vi "Sensor de Flujo.vi"() -> ()   [LabVIEW 2015]
uses:
  <vilib>/LabVIEW Interface for Arduino/Type Defs/Connection Type.ctl
  <vilib>/LabVIEW Interface for Arduino/Type Defs/Board Type.ctl
  <vilib>/LabVIEW Interface for Arduino/Type Defs/Pin Mode.ctl
  <vilib>/LabVIEW Interface for Arduino/LabVIEW Interface for Arduino.lvlib
  <vilib>/ptbypt/NI_PtbyPt.lvlib
panel:
  in  "Digital I/O Pin (0)":u8
  in  "VISA resource":refnum<visa-resource-name>
  out "LITROS POR MINUTO":dbl(graph)
  out "Horizontal Graduated Bar":dbl(slide) scale=0.0..100.0
  out "LITROS POR MINUTO 2":dbl(knob) scale=0.0..100.0
  out "Numeric":i32
  out "PULSOS POR SEGUNDO":i32
  out "CONTRO TIEMPO":dbl
  out "CONTEO":i32
  out "?":bool
  out "LITROS POR MINUTO":dbl
  out "?":string
  out "?":bool
  in  "?":bool
  # "MEDICIÓN DE FLUJO ATRAVEZ DEL SENSOR YF-S201"
  # "Militros/min"
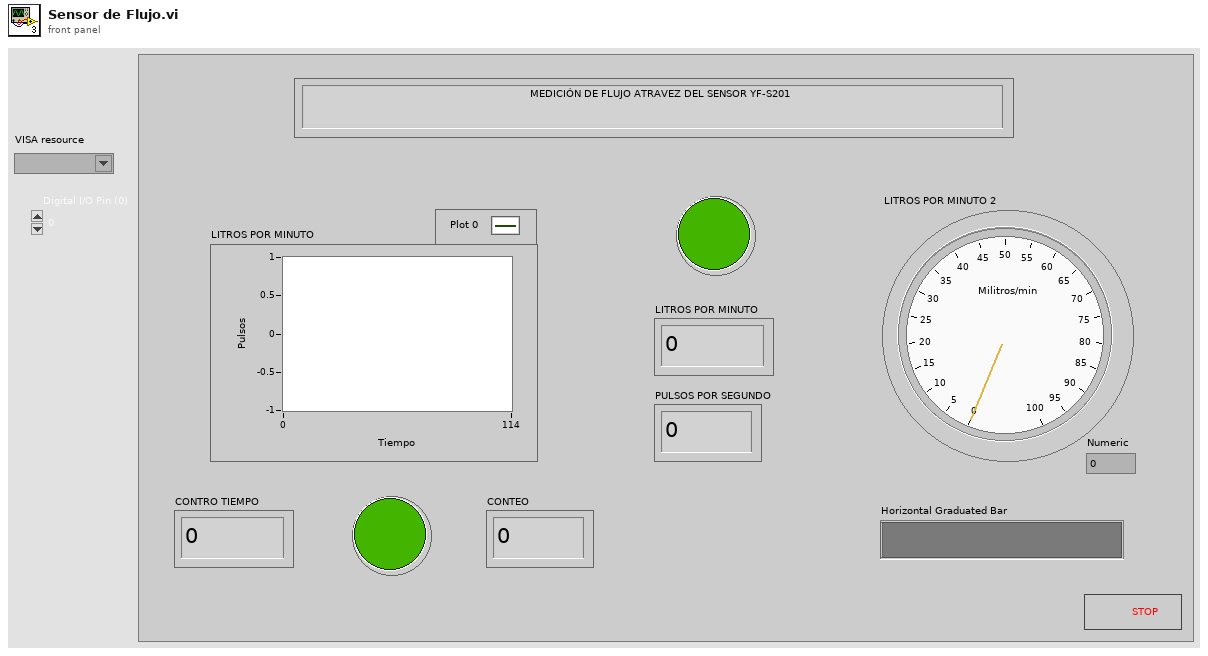
[diagram p1: front panel]
types:
  T1 = typedef "LabVIEW Interface for Arduino.lvlib/Board Type.ctl" = enum16{"Uno", "Dimuelanove w/Atmega 328", "Mega 2560"}
  T2 = typedef "LabVIEW Interface for Arduino.lvlib/Connection Type.ctl" = enum8{"USB / Serial", "XBEE", "BlueSmirf (Bluetooth)"}
  T3 = typedef "LabVIEW Interface for Arduino.lvlib/Arduino Resource.ctl" = cluster{"VISA resource":refnum<visa-resource-name>, "Board Type":T1, "Connection Type":enum8{"USB / Serial"}, "Bytes Per Packet (15)":u8}
  T4 = typedef "LabVIEW Interface for Arduino.lvlib/Pin Mode.ctl" = enum8{"Input", "Output"}
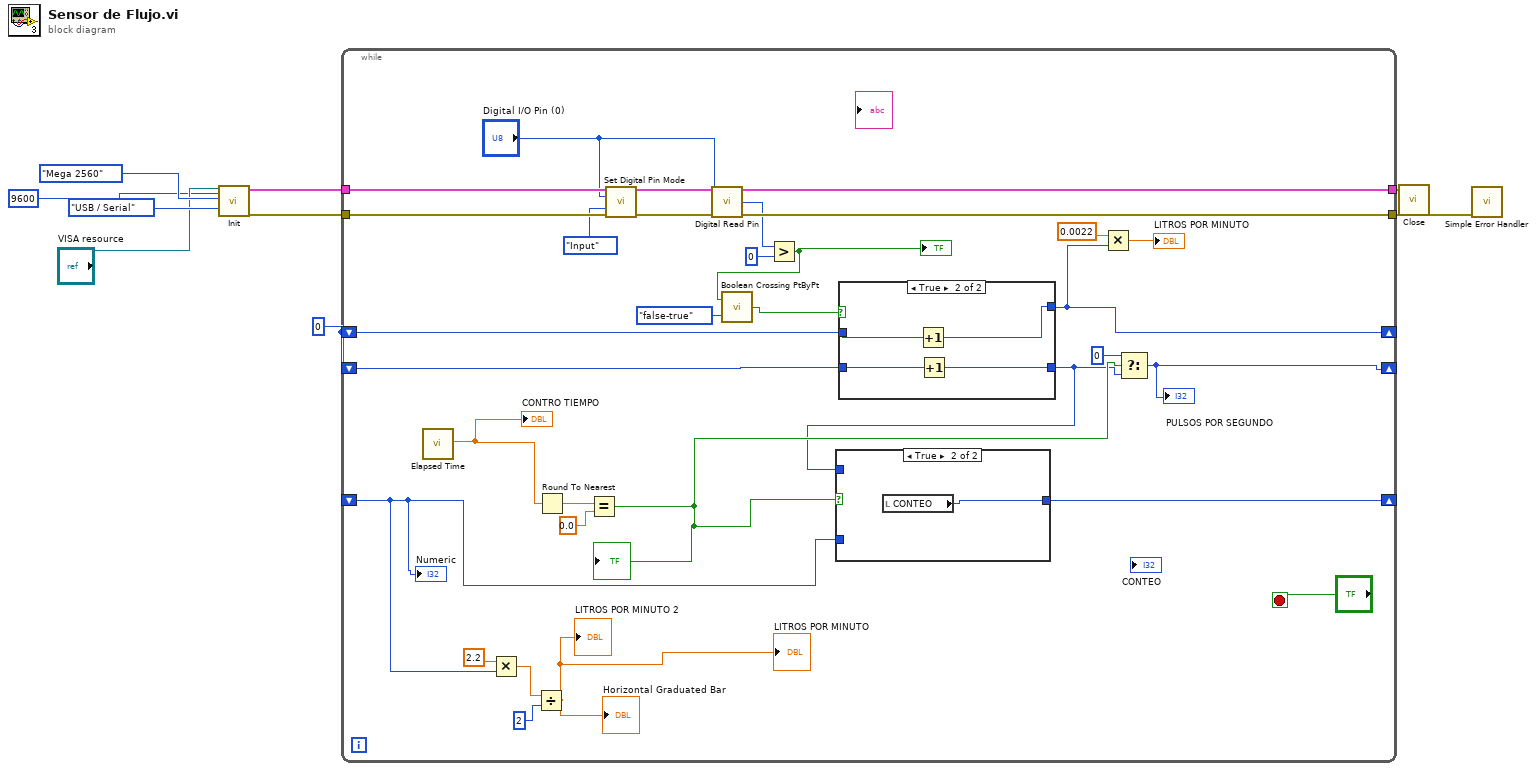
[diagram p0: block diagram]
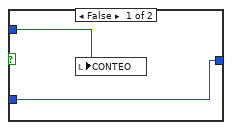
[diagram p2: hidden frame]
diagram:
  w3 = 0 ("CONTADOR 2")
  n1 = call <vilib>:"Init.vi"("VISA resource"="VISA resource", "Baud Rate (115200)"=u32 9600, "Board Type (Uno)"=Board_Type."Mega 2560", "Connection Type (USB/Serial)"=Connection_Type."USB / Serial") -> ("Arduino Resource"=w10:T3, "error out"=w9:errorcluster)  [unwired: 14 in]
  n2 = while {
    tunnel: w10 -> [w42]
    tunnel: w9 -> [w41]
    tunnel: [w34] -> w8
    tunnel: [w33] -> w6
    shift-right: [w30] -> _
    shift-left: w3 -> [w29]
    shift-right: [w20] -> _
    shift-left: w3 -> [w24]
    shift-right: [w19] -> _
    shift-left: _ -> [w16]
    stop <- "?" stop-if-true
    n3 = call "Elapsed Time"() -> ("Elapsed Time (s)"=w14:dbl)  [unwired: 12 in, 7 out]
    "CONTRO TIEMPO" <- w14
    n4 = Multiply(x=2.2, y=w16) -> (x*y=w15:dbl)
    n5 = Divide(x=w15, y=2) -> (x/y=→"LITROS POR MINUTO 2" →"Horizontal Graduated Bar" →"LITROS POR MINUTO":dbl)
    n6 = Round To Nearest(number=w14) -> (nearest integer value=w13:dbl)
    n7 = Equal?(x=w13, y=0.0) -> (x = y?=w22:bool)
    "?" <- w22
    n8 = call <vilib>:"Set Digital Pin Mode.vi"("Arduino Resource"=w42, "Digital I/O Pin"="Digital I/O Pin (0)", "Pin Mode (Input)"=Pin_Mode."Input", "error in"=w41) -> ("Arduino Resource"=w38:T3, "error out"=w37:errorcluster)  [unwired: 10 in]
    n9 = call <vilib>:"Digital Read Pin.vi"("Arduino Resource"=w38, "Digital I/O Pin (0)"="Digital I/O Pin (0)", "error in"=w37) -> ("Arduino Resource"=w34:T3, "Value"=w32:u8, "error out"=w33:errorcluster)  [unwired: 10 in]
    n10 = Greater?(x=w32, y=0) -> (0:w27:bool)
    "?" <- w27
    n11 = call <vilib>:"Boolean Crossing PtByPt.vi"("direction"=enum16{"either", "false-true", "true-false"}."false-true", "input"=w27) -> ("crossing"=w26:bool)  [unwired: 1 in]
    n12 = case shown="True" w26 {
      tunnel: [w47 w51] -> w30
      tunnel: w29 -> [w47 w50]
      tunnel: w24 -> [w46 w49]
      tunnel: [w46 w48] -> w21
      frame False {
      }
      frame True {
        n13 = Increment(x=w50) -> (x+1=w51:i32)
        n14 = Increment(x=w49) -> (x+1=w48:i32)
      }
    }
    n15 = case shown="True" w22 {
      tunnel: w21 -> [w44 _]
      tunnel: [w43 w45] -> w19
      tunnel: w16 -> [w43 _]
      frame False {
        n16 = local write "CONTEO"(w44) -> ()
      }
      frame True {
        n17 = local read "CONTEO"() -> (w45:i32)
      }
    }
    n18 = Multiply(x=0.0022, y=w30) -> (x*y=→"LITROS POR MINUTO":dbl)
    n19 = Select(t=0, s=w22, f=w21) -> (s? t:f=w20:i32)
    "PULSOS POR SEGUNDO" <- w20
    "Numeric" <- w16
  }
  n20 = call <vilib>:"Close.vi"("Arduino Resource"=w8, "error in"=w6) -> ("error out"=w7:errorcluster)  [unwired: 13 in]
  n21 = call <vilib>:"Simple Error Handler.vi"("error in (no error)"=w7) -> ()  [unwired: 4 in, 5 out]
